vi "ariLogger.vi"(9 "Input":string, 10 "Header":string="Begin Logging:\ncount,  constant,      OS Name,                  Laptop Ver,  Name,   Memory,       Disk, OS Ver") -> ()   [LabVIEW 2020]
doc: "Logs data to a new folder called \"logs\" within the directory that it is referenced in.\n\n\"Header\" is the first line used at the start of the logging.\n\n\"Input\" is the data that is written to each line. Can change line from line, only requirement is that it is a string.\n\nThis file does not run in a loop or have a wait to it, for usage look at testOfLogTesting.vi\n\nThis file does not format the header or data in any way, to automatically do that I have created stringHandler.vi"
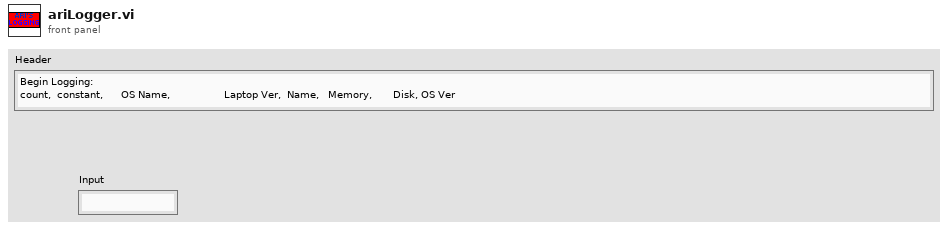
[diagram p1: front panel]
types:
  T1 = enum16{"open", "replace", "create", "open or create", "replace or create", "replace or create with confirmation"}
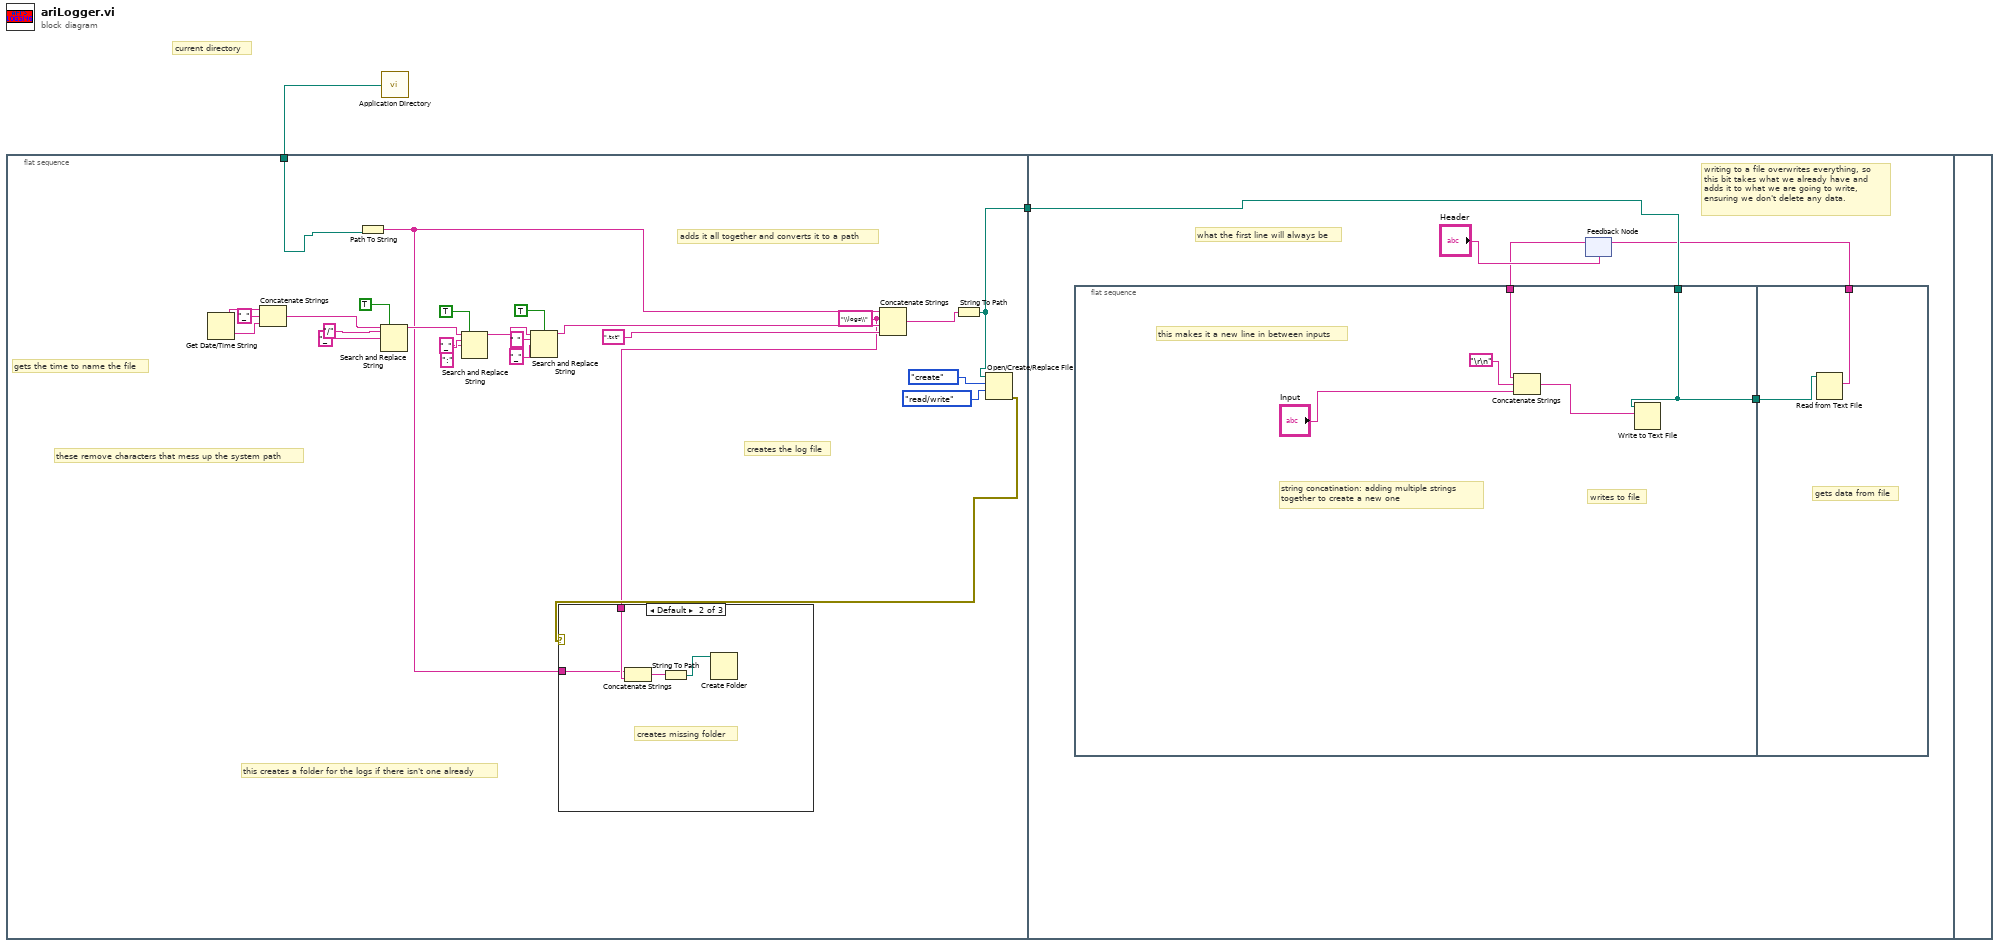
[diagram p0: block diagram]
diagram:
  # "current directory"
  n1 = flat-sequence {
    tunnel: [w9] -> w2
    tunnel: w1 -> [w6]
    tunnel: w2 -> [w35]
    frame #0 {
      w4 = "\\logs\\" ("string")
      # "adds it all together and converts it to a path"
      # "these remove characters that mess up the system path"
      # "gets the time to name the file"
      # "creates the log file"
      # "this creates a folder for the logs if there isn't one already"
      n2 = Get Date/Time String() -> (date string=w26:string, time string=w8:string)  [unwired: 3 in]
      n3 = Concatenate Strings(w26, "_" ("string"), w8) -> (w27:string)
      n4 = Path To String(path=w6) -> (string=w3:string)
      n5 = Search and Replace String(replace all?=TRUE ("replace all? (F)"), input string=w27, search string="/", replace string="_" ("replace string (\"\")")) -> (result string=w23:string)  [unwired: 4 in, 3 out]
      n6 = Search and Replace String(replace all?=TRUE ("replace all? (F)"), input string=w23, search string=":", replace string="_" ("replace string (\"\")")) -> (result string=w24:string)  [unwired: 4 in, 3 out]
      n7 = Search and Replace String(case sensitive?=TRUE ("ignore case? (F)"), input string=w24, search string=" ", replace string="_" ("replace string (\"\")")) -> (result string=w25:string)  [unwired: 4 in, 3 out]
      n8 = Concatenate Strings(w3, w4, w25, ".txt" ("string")) -> (w22:string)
      n9 = String To Path(string=w22) -> (path=w9:path)
      n10 = Open/Create/Replace File(file path (use dialog)=w9, operation (0:open)=T1."create", access (0:read/write)=enum16{"read/write", "read-only", "write-only"}."read/write") -> (error out=w5:errorcluster)  [unwired: 3 in, 2 out]
      n11 = case shown="Default" w5 {
        tunnel: w4 -> [_ w31 _]
        tunnel: w3 -> [_ w30 _]
        frame No Error {
        }
        frame Default {
          # "creates missing folder"
          n12 = Concatenate Strings(w30, w31) -> (w29:string)
          n13 = String To Path(string=w29) -> (path=w28:path)
          n14 = Create Folder(path (use dialog)=w28) -> ()  [unwired: 2 in, 3 out]
        }
        frame Error {
          # "actually able to run with this error"
        }
      }
    }
    frame #1 {
      # "writing to a file overwrites everything, so \nthis bit takes what we already have and \nadds it to what we are going to write, \nensuring we don't delete any data."
      # "what the first line will always be"
      n15 = flat-sequence {
        tunnel: w35 -> [w40]
        tunnel: [w40] -> w36
        tunnel: w33 -> [w37]
        tunnel: w36 -> [w43]
        tunnel: [w42] -> w32
        frame #0 {
          # "writes to file"
          # "string concatination: adding multiple strings\ntogether to create a new one"
          # "this makes it a new line in between inputs"
          n16 = Concatenate Strings(w37, "\r\n", "Input") -> (w41:string)
          n17 = Write to Text File(file (use dialog)=w40, text=w41) -> ()  [unwired: 2 in, 3 out]
        }
        frame #1 {
          # "gets data from file"
          n18 = Read from Text File(file (use dialog)=w43) -> (text=w42:string)  [unwired: 3 in, 3 out]
        }
      }
      n19 = feedback-in #1(w32) -> ()
      n20 = feedback #1("Header") -> (w33:string)
    }
    frame #2 {
    }
  }
  n21 = call <vilib>:"Application Directory.vi"() -> ("Application Directory"=w1:path)
